vi "SerialRead.vi"() -> ()   [LabVIEW 2013]
uses:
  <vilib>/Instr/_visa.llb/VISA Configure Serial Port (Instr).vi
panel:
  out "unsigned byte array 2":u8[](array[numeric])
  out "unsigned byte array":u8[](array[numeric])
  in  "stop":bool
  in  "serial_port":refnum<visa-resource-name> caption="Porta Serial"
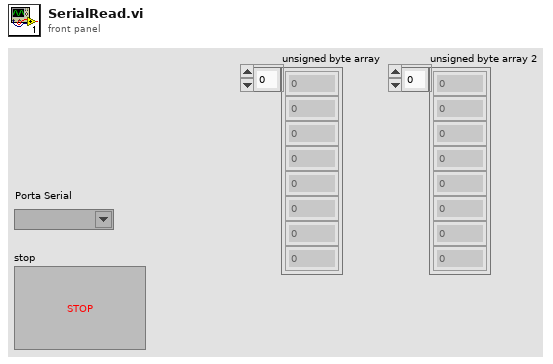
[diagram p1: front panel]
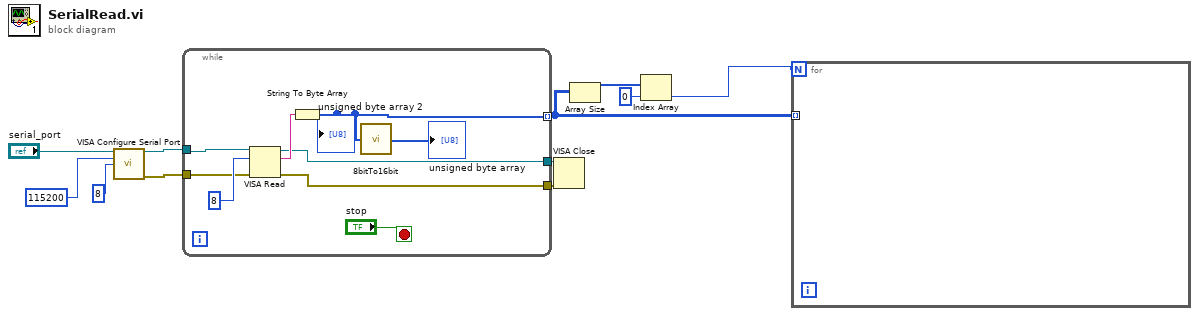
[diagram p0: block diagram]
diagram:
  n1 = call-poly "VISA Configure Serial Port"("VISA resource name"="serial_port", "baud rate (9600)"=u32 115200, "data bits (8)"=u16 8) -> ("VISA resource name out"=w8:refnum<visa-resource-name>, "error out"=w7:errorcluster)  [unwired: 11 in]
  n2 = while {
    tunnel: w8 -> [w19]
    tunnel: w7 -> [w18]
    tunnel: [w16] -> w6
    tunnel: [w15] -> w5
    tunnel: [w13] -> w4 mode=indexing
    stop <- "stop" stop-if-true
    n3 = VISA Read(VISA resource name=w19, byte count=u32 8, error in (no error)=w18) -> (VISA resource name out=w15:refnum<visa-resource-name>, read buffer=w17:string, error out=w16:errorcluster)  [unwired: 1 out]
    n4 = String To Byte Array(string=w17) -> (unsigned byte array=w13:u8[])
    "unsigned byte array 2" <- w13
    n5 = call "8bitTo16bit.vi"("input_byte"=w13) -> ("output_int16"=→"unsigned byte array":i32[])
  }
  n6 = VISA Close(VISA resource name=w5, error in (no error)=w6) -> ()  [unwired: 1 out]
  n7 = Array Size(array=w4) -> (size(s)=w3:i32[])
  n8 = Index Array(array=w3, index=0) -> (element=w1:i32)
  n9 = for {
    N: w1 -> [_]
    tunnel: w4 -> [_] mode=indexing
  }
